vi "CrioLinux.vi"() -> ()   [LabVIEW 2017]
uses:
  <vilib>/rvi/Emulation/niFpgaGetClockAttributes.vi
  <vilib>/rvi/Emulation/niFpgaSctlEmulationGetInTimedLoop.vi
  <vilib>/rvi/Emulation/niFpgaEmulationReportErrorSimple.vi
  <vilib>/rvi/eio/common/nirviEmuTemplateMethod_errors.vi
  <vilib>/rvi/Emulation/niFpgaCriticalErrorInLSC.vi
  <vilib>/eio/EIONode/EIONode.xnode
panel:
  in  "Mod3/DIO31":bool
  in  "Mod2/DIO0":bool
  in  "Mod2/DIO1":bool
  in  "Mod2/DIO2":bool
  in  "Mod2/DIO3":bool
  in  "Mod2/DIO4":bool
  in  "Mod2/DIO5":bool
  in  "Mod2/DIO6":bool
  in  "Mod2/DIO7":bool
  in  "Mod1/DIO0":bool
  in  "Mod1/DIO1":bool
  in  "Mod1/DIO2":bool
  in  "Mod1/DIO3":bool
  in  "Mod1/DIO4":bool
  in  "Mod1/DIO5":bool
  in  "Mod1/DIO6":bool
  in  "Mod1/DIO7":bool
  out "Mod3/DIO":u64
  out "Mod4/AI3":sgl
  out "Mod4/AI2":sgl
  out "Mod4/AI1":sgl
  out "Mod4/AI0":sgl
  in  "Mod5/AO0":sgl
  in  "Mod5/AO1":sgl
  in  "Mod5/AO2":sgl
  in  "Mod5/AO3":sgl
  out "Mod6/TC3":sgl
  out "Mod6/TC2":sgl
  out "Mod6/TC1":sgl
  out "Mod6/TC0":sgl
  out "Mod7/AI3":sgl
  out "Mod7/AI2":sgl
  out "Mod7/AI1":sgl
  out "Mod7/AI0":sgl
  out "Mod8/AI0":sgl
  out "Mod8/AI1":sgl
  out "Mod8/AI2":sgl
  out "Mod8/AI3":sgl
  # "Binary inputs"
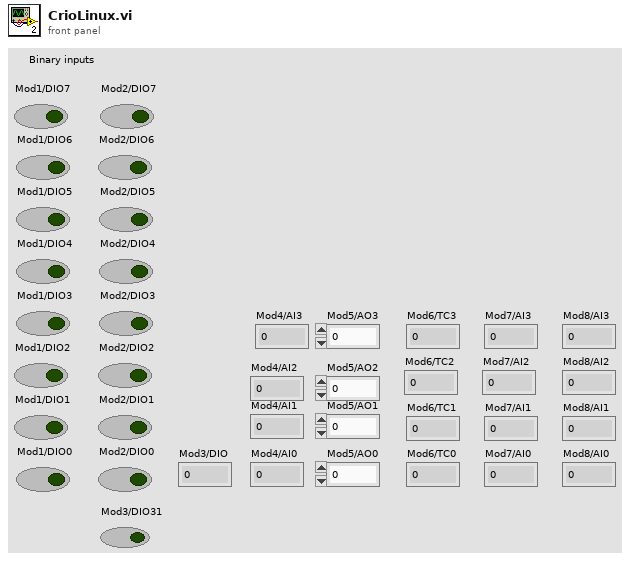
[diagram p1: front panel]
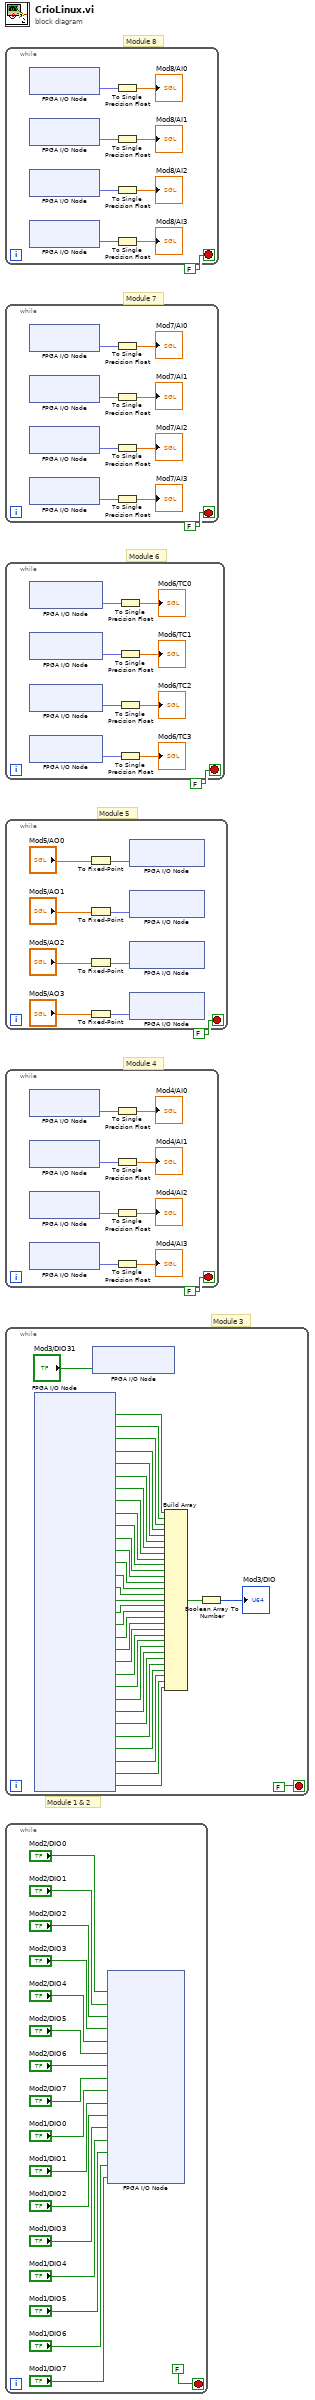
[diagram p0: block diagram]
diagram:
  # "Module 1 & 2"
  # "Module 3"
  # "Module 4"
  # "Module 5"
  # "Module 6"
  # "Module 7"
  # "Module 8"
  n1 = while {
    stop <- FALSE stop-if-true
    n2 = xnode "FPGA I/O Node"() -> ("Mod8/AI0"=w6:fxp<+/-,20,5>)  [unwired: 1 in, 1 out]
    n3 = xnode "FPGA I/O Node"() -> ("Mod8/AI1"=w4:fxp<+/-,20,5>)  [unwired: 1 in, 1 out]
    n4 = xnode "FPGA I/O Node"() -> ("Mod8/AI2"=w2:fxp<+/-,20,5>)  [unwired: 1 in, 1 out]
    n5 = xnode "FPGA I/O Node"() -> ("Mod8/AI3"=w8:fxp<+/-,20,5>)  [unwired: 1 in, 1 out]
    n6 = To Single Precision Float(number=w6) -> (single precision float=→"Mod8/AI0":sgl)
    n7 = To Single Precision Float(number=w4) -> (single precision float=→"Mod8/AI1":sgl)
    n8 = To Single Precision Float(number=w2) -> (single precision float=→"Mod8/AI2":sgl)
    n9 = To Single Precision Float(number=w8) -> (single precision float=→"Mod8/AI3":sgl)
  }
  n10 = while {
    stop <- FALSE stop-if-true
    n11 = xnode "FPGA I/O Node"() -> ("Mod7/AI0"=w15:fxp<+/-,20,5>)  [unwired: 1 in, 1 out]
    n12 = xnode "FPGA I/O Node"() -> ("Mod7/AI1"=w13:fxp<+/-,20,5>)  [unwired: 1 in, 1 out]
    n13 = xnode "FPGA I/O Node"() -> ("Mod7/AI2"=w11:fxp<+/-,20,5>)  [unwired: 1 in, 1 out]
    n14 = xnode "FPGA I/O Node"() -> ("Mod7/AI3"=w17:fxp<+/-,20,5>)  [unwired: 1 in, 1 out]
    n15 = To Single Precision Float(number=w15) -> (single precision float=→"Mod7/AI0":sgl)
    n16 = To Single Precision Float(number=w13) -> (single precision float=→"Mod7/AI1":sgl)
    n17 = To Single Precision Float(number=w11) -> (single precision float=→"Mod7/AI2":sgl)
    n18 = To Single Precision Float(number=w17) -> (single precision float=→"Mod7/AI3":sgl)
  }
  n19 = while {
    stop <- FALSE stop-if-true
    n20 = xnode "FPGA I/O Node"() -> ("Mod6/TC0"=w24:fxp<+/-,24,-2>)  [unwired: 1 in, 1 out]
    n21 = xnode "FPGA I/O Node"() -> ("Mod6/TC1"=w22:fxp<+/-,24,-2>)  [unwired: 1 in, 1 out]
    n22 = xnode "FPGA I/O Node"() -> ("Mod6/TC2"=w20:fxp<+/-,24,-2>)  [unwired: 1 in, 1 out]
    n23 = xnode "FPGA I/O Node"() -> ("Mod6/TC3"=w26:fxp<+/-,24,-2>)  [unwired: 1 in, 1 out]
    n24 = To Single Precision Float(number=w24) -> (single precision float=→"Mod6/TC0":sgl)
    n25 = To Single Precision Float(number=w22) -> (single precision float=→"Mod6/TC1":sgl)
    n26 = To Single Precision Float(number=w20) -> (single precision float=→"Mod6/TC2":sgl)
    n27 = To Single Precision Float(number=w26) -> (single precision float=→"Mod6/TC3":sgl)
  }
  n28 = while {
    stop <- FALSE stop-if-true
    n29 = To Fixed-Point(number="Mod5/AO0") -> (fixed-point=w35:fxp<+/-,20,5>)  [unwired: 1 in]
    n30 = To Fixed-Point(number="Mod5/AO1") -> (fixed-point=w34:fxp<+/-,20,5>)  [unwired: 1 in]
    n31 = To Fixed-Point(number="Mod5/AO2") -> (fixed-point=w33:fxp<+/-,20,5>)  [unwired: 1 in]
    n32 = To Fixed-Point(number="Mod5/AO3") -> (fixed-point=w32:fxp<+/-,20,5>)  [unwired: 1 in]
    n33 = xnode "FPGA I/O Node"("Mod5/AO0"=w35) -> ()  [unwired: 1 in, 1 out]
    n34 = xnode "FPGA I/O Node"("Mod5/AO1"=w34) -> ()  [unwired: 1 in, 1 out]
    n35 = xnode "FPGA I/O Node"("Mod5/AO2"=w33) -> ()  [unwired: 1 in, 1 out]
    n36 = xnode "FPGA I/O Node"("Mod5/AO3"=w32) -> ()  [unwired: 1 in, 1 out]
  }
  n37 = while {
    stop <- FALSE stop-if-true
    n38 = xnode "FPGA I/O Node"() -> ("Mod4/AI0"=w42:fxp<+/-,20,5>)  [unwired: 1 in, 1 out]
    n39 = xnode "FPGA I/O Node"() -> ("Mod4/AI1"=w40:fxp<+/-,20,5>)  [unwired: 1 in, 1 out]
    n40 = xnode "FPGA I/O Node"() -> ("Mod4/AI2"=w38:fxp<+/-,20,5>)  [unwired: 1 in, 1 out]
    n41 = xnode "FPGA I/O Node"() -> ("Mod4/AI3"=w44:fxp<+/-,20,5>)  [unwired: 1 in, 1 out]
    n42 = To Single Precision Float(number=w42) -> (single precision float=→"Mod4/AI0":sgl)
    n43 = To Single Precision Float(number=w40) -> (single precision float=→"Mod4/AI1":sgl)
    n44 = To Single Precision Float(number=w38) -> (single precision float=→"Mod4/AI2":sgl)
    n45 = To Single Precision Float(number=w44) -> (single precision float=→"Mod4/AI3":sgl)
  }
  n46 = while {
    stop <- FALSE stop-if-true
    n47 = xnode "FPGA I/O Node"() -> ("Mod3/DIO0"=w80:bool, "Mod3/DIO1"=w79:bool, "Mod3/DIO2"=w76:bool, "Mod3/DIO3"=w75:bool, "Mod3/DIO4"=w74:bool, "Mod3/DIO5"=w73:bool, "Mod3/DIO6"=w72:bool, "Mod3/DIO7"=w71:bool, "Mod3/DIO8"=w70:bool, "Mod3/DIO9"=w69:bool, "Mod3/DIO10"=w68:bool, "Mod3/DIO11"=w67:bool, "Mod3/DIO12"=w66:bool, "Mod3/DIO13"=w65:bool, "Mod3/DIO14"=w64:bool, "Mod3/DIO15"=w63:bool, "Mod3/DIO16"=w61:bool, "Mod3/DIO17"=w60:bool, "Mod3/DIO18"=w59:bool, "Mod3/DIO19"=w58:bool, "Mod3/DIO20"=w57:bool, "Mod3/DIO21"=w56:bool, "Mod3/DIO22"=w55:bool, "Mod3/DIO23"=w54:bool, "Mod3/DIO24"=w53:bool, "Mod3/DIO25"=w52:bool, "Mod3/DIO26"=w51:bool, "Mod3/DIO27"=w50:bool, "Mod3/DIO28"=w49:bool, "Mod3/DIO29"=w48:bool, "Mod3/DIO30"=w47:bool)  [unwired: 31 in, 31 out]
    n48 = xnode "FPGA I/O Node"("Mod3/DIO31"="Mod3/DIO31") -> ()  [unwired: 1 in, 1 out]
    n49 = Build Array(w80, w79, w76, w75, w74, w73, w72, w71, w70, w69, w68, w67, w66, w65, w64, w63, w61, w60, w59, w58, w57, w56, w55, w54, w53, w52, w51, w50, w49, w48, w47) -> (w62:bool[])
    n50 = Boolean Array To Number(Boolean array=w62) -> (number=→"Mod3/DIO":u64)
  }
  n51 = while {
    stop <- FALSE stop-if-true
    n52 = xnode "FPGA I/O Node"("Mod2/DIO0"="Mod2/DIO0", "Mod2/DIO1"="Mod2/DIO1", "Mod2/DIO2"="Mod2/DIO2", "Mod2/DIO3"="Mod2/DIO3", "Mod2/DIO4"="Mod2/DIO4", "Mod2/DIO5"="Mod2/DIO5", "Mod2/DIO6"="Mod2/DIO6", "Mod2/DIO7"="Mod2/DIO7", "Mod1/DIO0"="Mod1/DIO0", "Mod1/DIO1"="Mod1/DIO1", "Mod1/DIO2"="Mod1/DIO2", "Mod1/DIO3"="Mod1/DIO3", "Mod1/DIO4"="Mod1/DIO4", "Mod1/DIO5"="Mod1/DIO5", "Mod1/DIO6"="Mod1/DIO6", "Mod1/DIO7"="Mod1/DIO7") -> ()  [unwired: 16 in, 16 out]
  }
